vi "Y Limiter_ext.vi"(5 "reinitialize? (F)":bool, 6 "Y_limiter_old":T1 {"output" format="%.2f"}, 7 "X1(SetState)":T3(ring)=enum."max", 9 "Y param":T4={"output high"=100.0, "alr value"=0.0, "output low"=0.0, "output time (t)"=1.0} {"output time (t)" format="%.2f"; "output low" format="%.3f"; "alr value" format="%.3f"; "output high" format="%.3f"}, 10 "Y (NaN)":dbl=nan, 11 "Y_Set":dbl) -> (1 "End":bool, 2 "SpLim_State":T2=enum."increase", 3 "output":dbl format="%.2f", 4 "Y_limiter":T1 {"output" format="%.2f"})   [LabVIEW 2019, in "control.lvlib"]
uses:
  control.lvlib
  ctl/control param simple.ctl
  ctl/Y_Lim_State.ctl
  ctl/Y_Lim_ext_defs.ctl
  PID/PID Timing Estimation Ext.vi
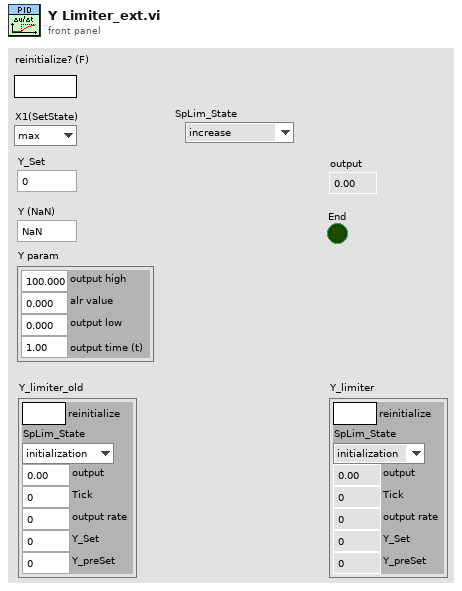
[diagram p1: front panel]
types:
  T1 = typedef "control.lvlib/Y_Lim_ext_defs.ctl" = cluster{"reinitialize":bool, "SpLim_State":T2, "output":dbl, "Tick":u32, "output rate":dbl, "Y_Set":dbl, "Y_preSet":dbl}
  T2 = typedef "control.lvlib/Y_Lim_State.ctl" = enum8{"initialization", "alarm", "stop", "decrease", "increase"}
  T3 = enum8{"alarm", "min", "stop", "hand", "auto", "max"}
  T4 = typedef "control.lvlib/control param simple.ctl" = cluster{"output high":dbl, "alr value":dbl, "output low":dbl, "output time (t)":dbl}
  T5 = cluster{bool, "SpLim_State":T2, "output":dbl, "Tick":u32, "output rate":dbl, "output high":dbl, "Y_preSet":dbl}
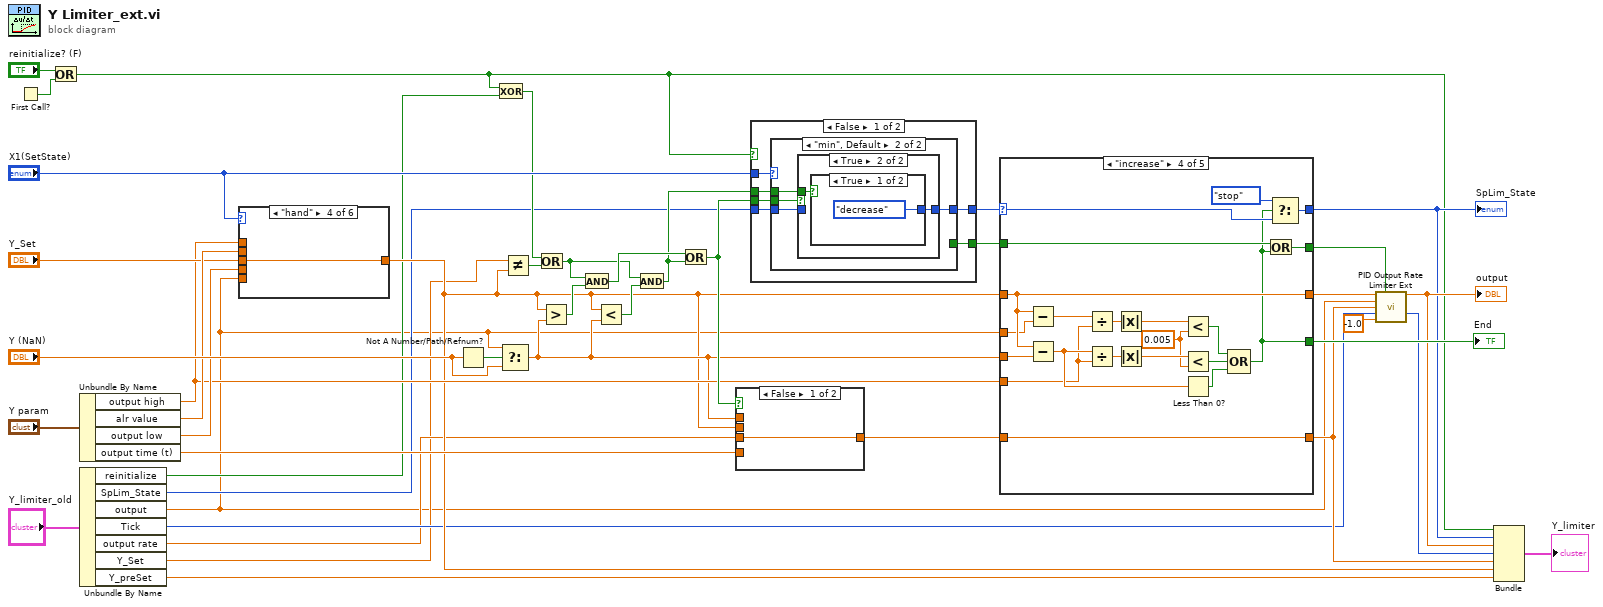
[diagram p0: block diagram]
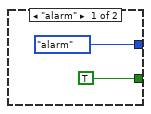
[diagram p7: hidden frame]
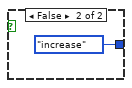
[diagram p9: hidden frame]
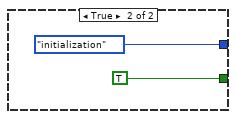
[diagram p10: hidden frame]
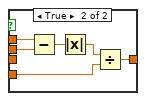
[diagram p11: hidden frame]
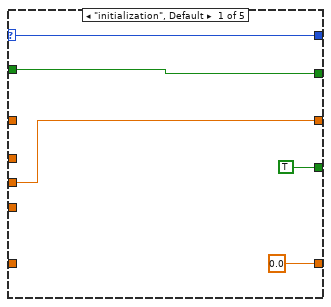
[diagram p12: hidden frame]
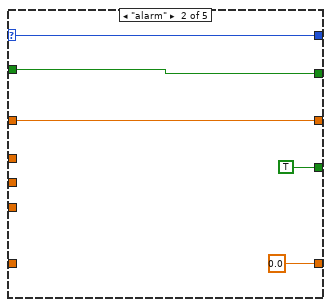
[diagram p13: hidden frame]
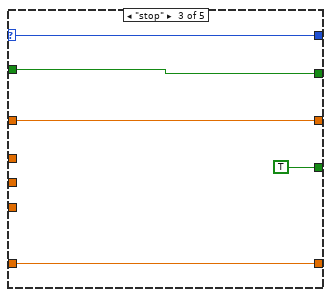
[diagram p14: hidden frame]
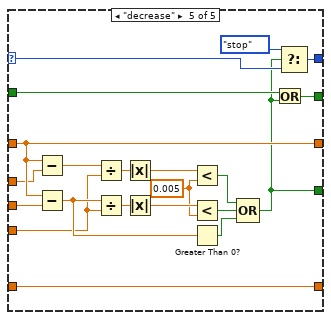
[diagram p15: hidden frame]
diagram:
  n1 = First Call?() -> (First Call?: T/F=w28:bool)
  n2 = Or(x="reinitialize? (F)", y=w28) -> (x .or. y?=w9:bool)
  n3 = Unbundle By Name("Y param") -> ("output high"=w19:dbl, "alr value"=w27:dbl, "output low"=w26:dbl, "output time (t)"=w38:dbl)
  n4 = Unbundle By Name("Y_limiter_old") -> ("reinitialize"=w7:bool, "SpLim_State"=w6:T2, "output"=w1:dbl, "Tick"=w5:u32, "output rate"=w4:dbl, "Y_Set"=w3:dbl, "Y_preSet"=w2:dbl)
  n5 = case shown="\"hand\"" "X1(SetState)" {
    tunnel: w19 -> [_ _ _ _ _ w48]
    tunnel: w27 -> [w43 _ _ _ _ _]
    tunnel: w26 -> [_ w44 _ _ _ _]
    tunnel: "Y_Set" -> [_ _ _ w46 w47 _]
    tunnel: [w43 w44 w45 w46 w47 w48] -> w11
    tunnel: w1 -> [_ _ w45 _ _ _]
    frame "alarm", Default {
    }
    frame "min" {
    }
    frame "stop" {
    }
    frame "hand" {
    }
    frame "auto" {
    }
    frame "max" {
    }
  }
  n6 = Not A Number/Path/Refnum?(number/path/refnum="Y (NaN)") -> (NaN/Path/Refnum?=w35:bool)
  n7 = Exclusive Or(1:w7, 2:w9) -> (0:w17:bool)
  n8 = Select(t=w1, s=w35, f="Y (NaN)") -> (s? t:f=w16:dbl)
  n9 = Not Equal?(x=w3, y=w11) -> (x != y?=w31:bool)
  n10 = Or(x=w17, y=w31) -> (x .or. y?=w18:bool)
  n11 = Greater?(x=w11, y=w16) -> (0:w33:bool)
  n12 = And(x=w18, y=w33) -> (x .and. y?=w32:bool)
  n13 = Less?(x=w11, y=w16) -> (x < y?=w30:bool)
  n14 = And(x=w18, y=w30) -> (x .and. y?=w23:bool)
  n15 = Or(x=w32, y=w23) -> (x .or. y?=w24:bool)
  n16 = case shown="False" w24 {
    tunnel: w16 -> [_ w50]
    tunnel: w11 -> [_ w51]
    tunnel: w4 -> [w49 _]
    tunnel: [w49 w53] -> w36
    tunnel: w38 -> [_ w52]
    frame False {
    }
    frame True {
      n17 = Subtract(x=w50, y=w51) -> (x-y=w54:dbl)
      n18 = Absolute Value(x=w54) -> (abs(x)=w55:dbl)
      n19 = Divide(x=w55, y=w52) -> (x/y=w53:dbl)
    }
  }
  n20 = case shown="False" w9 {
    tunnel: [w60 Y_Lim_State."initialization" ("SpLim_State")] -> w22
    tunnel: [w56 TRUE] -> w20
    tunnel: w24 -> [w61 _]
    tunnel: w23 -> [w59 _]
    tunnel: w6 -> [w58 _]
    tunnel: "X1(SetState)" -> [w57 _]
    frame False {
      n21 = case shown="\"min\", Default" w57 {
        tunnel: w61 -> [_ w67]
        tunnel: [Y_Lim_State."alarm" ("SpLim_State") w66] -> w60
        tunnel: w59 -> [_ w65]
        tunnel: w58 -> [_ w64]
        tunnel: [TRUE _] -> w56
        frame "alarm" {
        }
        frame "min", Default {
          n22 = case shown="True" w67 {
            tunnel: [w68 w70] -> w66
            tunnel: w65 -> [_ w69]
            tunnel: w64 -> [w68 _]
            frame False {
            }
            frame True {
              n23 = case shown="True" w69 {
                tunnel: [Y_Lim_State."decrease" ("SpLim_State") Y_Lim_State."increase" ("SpLim_State")] -> w70
                frame True {
                }
                frame False {
                }
              }
            }
          }
        }
      }
    }
    frame True {
    }
  }
  n24 = case shown="\"increase\"" w22 {
    selector: w22 -> [w75 w80 w87 w103 w124]
    tunnel: w11 -> [_ w81 w88 w101 w122]
    tunnel: w16 -> [w77 _ _ w96 w117]
    tunnel: [w77 w81 w88 w101 w122] -> w39
    tunnel: [TRUE TRUE TRUE w90 w111] -> w42
    tunnel: [0.0 0.0 w86 w106 w127] -> w12
    tunnel: [w76 w82 w85 w91 w113] -> w41
    tunnel: [w75 w80 w87 w104 w125] -> w10
    tunnel: w36 -> [_ _ w86 w106 w127]
    tunnel: w1 -> [_ _ _ w100 w121]
    tunnel: w19 -> [_ _ _ w94 w115]
    tunnel: w20 -> [w76 w82 w85 w92 w112]
    frame "initialization", Default {
    }
    frame "alarm" {
    }
    frame "stop" {
    }
    frame "increase" {
      w93 = 0.005 ("y")
      n25 = Subtract(x=w101, y=w100) -> (x-y=w97:dbl)
      n26 = Subtract(x=w101, y=w96) -> (x-y=w105:dbl)
      n27 = Divide(x=w97, y=w94) -> (x/y=w98:dbl)
      n28 = Divide(x=w105, y=w94) -> (x/y=w110:dbl)
      n29 = Absolute Value(x=w98) -> (abs(x)=w99:dbl)
      n30 = Absolute Value(x=w110) -> (abs(x)=w109:dbl)
      n31 = Less?(x=w99, y=w93) -> (x < y?=w95:bool)
      n32 = Less?(x=w109, y=w93) -> (x < y?=w108:bool)
      n33 = Less Than 0?(x=w105) -> (x < 0?=w107:bool)
      n34 = Compound Arithmetic op=OR(w95, w108, w107) -> (w90:bool)
      n35 = Or(x=w92, y=w90) -> (x .or. y?=w91:bool)
      n36 = Select(t=Y_Lim_State."stop", s=w90, f=w103) -> (s? t:f=w104:T2)
    }
    frame "decrease" {
      w114 = 0.005 ("y")
      n37 = Subtract(x=w122, y=w121) -> (x-y=w118:dbl)
      n38 = Subtract(x=w122, y=w117) -> (x-y=w126:dbl)
      n39 = Divide(x=w118, y=w115) -> (x/y=w119:dbl)
      n40 = Divide(x=w126, y=w115) -> (x/y=w131:dbl)
      n41 = Absolute Value(x=w119) -> (abs(x)=w120:dbl)
      n42 = Absolute Value(x=w131) -> (abs(x)=w130:dbl)
      n43 = Less?(x=w120, y=w114) -> (x < y?=w116:bool)
      n44 = Less?(x=w130, y=w114) -> (x < y?=w129:bool)
      n45 = Greater Than 0?(x=w126) -> (x > 0?=w128:bool)
      n46 = Compound Arithmetic op=OR(w116, w129, w128) -> (w111:bool)
      n47 = Or(x=w112, y=w111) -> (x .or. y?=w113:bool)
      n48 = Select(t=Y_Lim_State."stop", s=w111, f=w124) -> (s? t:f=w125:T2)
    }
  }
  "End" <- w42
  "SpLim_State" <- w10
  n49 = call "PID Output Rate Limiter Ext.vi"("input (controller output)"=w39, "reinitialize? (F)"=w41, "output old"=w1, "output rate (EGU/s)"=w12, "Tick old"=w5, "dt (s)"=-1.0) -> ("output"=w14:dbl, "Tick"=w13:u32)  [unwired: 7 in, 1 out]
  "output" <- w14
  n50 = Bundle(w9, "SpLim_State"=w10, "output"=w14, "Tick"=w13, "output rate"=w12, "output high"=w11, "Y_preSet"=w2) -> (→"Y_limiter":T5)  [unwired: 1 in]
